vi "check_valve_status.vi"(11 "Channel 1":tag) -> (1 "Ch. 3 value":dbl format="%0.2f", 2 "Ch. 2 value":dbl format="%0.2f", 3 "Ch. 1 value":dbl format="%0.2f")   [LabVIEW 2014]
uses:
  <vilib>/DAQmx/create/channels.llb/DAQmx Create Channel (AI-Voltage-Basic).vi
  <vilib>/DAQmx/read.llb/DAQmx Read (Analog 1D DBL NChan 1Samp).vi
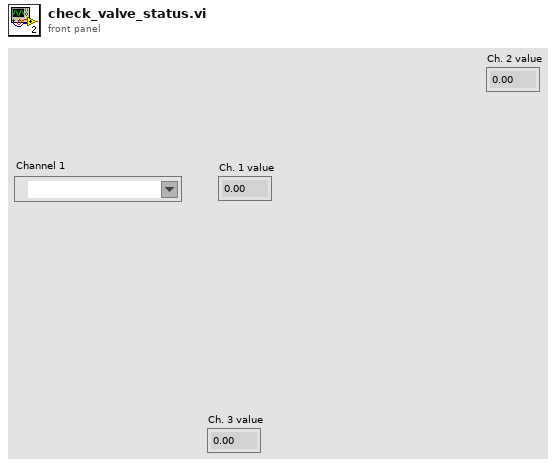
[diagram p1: front panel]
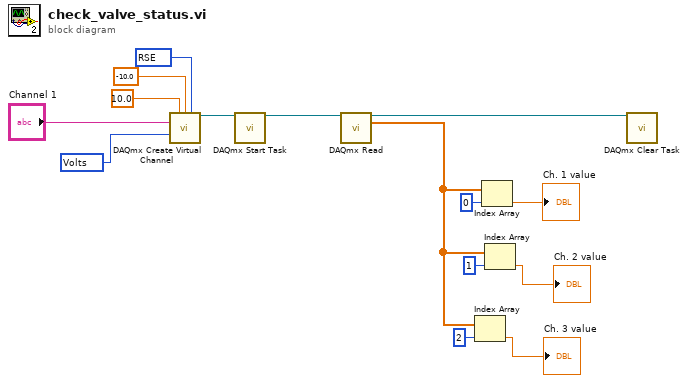
[diagram p0: block diagram]
diagram:
  w8 = 10083 items=["default"=-1, "RSE"=10083, "NRSE"=10078, "Differential"=10106, "Pseudodifferential"=12529] ("input terminal configuration")
  w11 = 10348 items=["Volts"=10348, "From Custom Scale"=10065] ("units")
  n1 = call-poly <vilib>:"DAQmx Create Virtual Channel.vi"("maximum value"=10.0, "minimum value"=-10.0, "input terminal configuration"=w8, "physical channels"="Channel 1", "units"=w11) -> ("task out"=w10:refnum<k21>)  [unwired: 9 in, 1 out]
  n2 = call <vilib>:"DAQmx Start Task.vi"("task/channels in"=w10) -> ("task out"=w9:refnum<k21>)  [unwired: 13 in, 1 out]
  n3 = call-poly <vilib>:"DAQmx Read.vi"("task/channels in"=w9) -> ("task out"=w14:refnum<k21>, "data"=w1:dbl[])  [unwired: 12 in, 1 out]
  n4 = Index Array(array=w1, index=2) -> (element=→"Ch. 3 value":dbl)
  n5 = Index Array(array=w1, index=0) -> (element=→"Ch. 1 value":dbl)
  n6 = Index Array(array=w1, index=1) -> (element=→"Ch. 2 value":dbl)
  n7 = call <vilib>:"DAQmx Clear Task.vi"("task in"=w14) -> ()  [unwired: 14 in, 1 out]
